vi "test Convert String To 9403 Module.vi"(8 "error in (no error)":errorcluster, 11 "TestCase in":refnum<class "RSI Module Unit Tests.lvclass">) -> (0 "error out":errorcluster, 3 "TestCase out":refnum<class "RSI Module Unit Tests.lvclass">)   [LabVIEW 2017, in "RSI Module Unit Tests.lvclass"]
uses:
  RSI Module Unit Tests.lvclass
  RSI Module/Module Models.ctl
  RSI Module/Slot Settings.ctl
  <vilib>/addons/_JKI Toolkits/VI Tester/TestCase.llb/TestCase.lvclass
  RSI Module/RSI Module.lvclass
  C:/Program Files (x86)/National Instruments/LabVIEW 2017/vi.lib/addons/_JKI Toolkits/VI Tester/TestCase.llb/TestCase.lvclass
panel:
  in  "xml string":string="<Object>\r\n<Name>RSI Module out</Name>\r\n<NumLevels>2</NumLevels>\r\n<Class>Modules.lvlib:9403.lvclass</Class>\r\n<Version>1.0.0.1</Version>\r\n<Version>1.0.0.21</Version>\r\n<Cluster>\r\n<Name>RSI Module.lvclass</Name>\r\n<NumElts>3</NumElts>\r\n<String>\r\n<Name>Module</Name>\r\n<Val>NI 9403</Val>\r\n</String>\r\n<Cluster>\r\n<Name>Slot Settings</Name>\r\n<NumElts>2</NumElts>\r\n<U32>\r\n<Name>Slot</Name>\r\n<Val>1</Val>\r\n</U32>\r\n<Boolean>\r\n<Name>EtherCAT?</Name>\r\n<Val>1</Val>\r\n</Boolean>\r\n</Cluster>\r\n<Cluster>\r\n<Name>Channels</Name>\r\n<NumElts>4</NumElts>\r\n<I32>\r\n<Name># Input Channels</Name>\r\n<Val>32</Val>\r\n</I32>\r\n<I32>\r\n<Name># Output Channels</Name>\r\n<Val>0</Val>\r\n</I32>\r\n<EW>\r\n<Name>Channel Type</Name>\r\n<Choice>Analog</Choice>\r\n<Choice>Digital</Choice>\r\n<Val>1</Val>\r\n</EW>\r\n<String>\r\n<Name>Units</Name>\r\n<Val></Val>\r\n</String>\r\n</Cluster>\r\n</Cluster>\r\n<Cluster>\r\n</Cluster>\r\n</Object>\r\n"
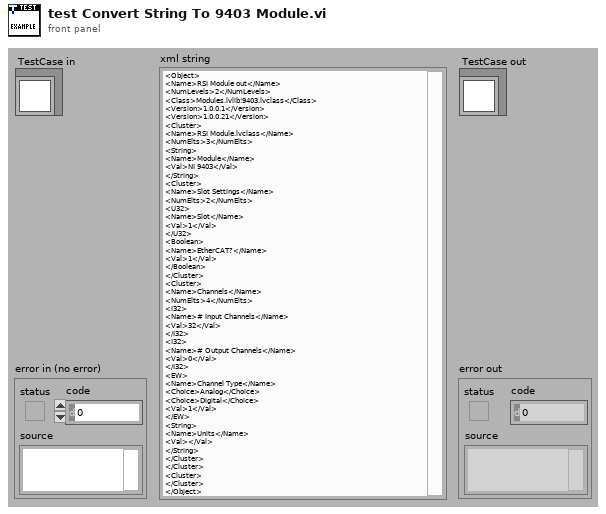
[diagram p1: front panel]
types:
  T1 = typedef "Modules.lvlib/RSI Module.lvclass/Slot Settings.ctl" = cluster{"Slot":u32, "EtherCAT?":bool}
  T2 = typedef "Modules.lvlib/RSI Module.lvclass/Module Models.ctl" = enum16{"Empty", "NI 9201", "NI 9203", "NI 9205", "NI 9206", "NI 9207", "NI 9208", "NI 9211", "NI 9212", "NI 9213", "NI 9214", "NI 9215", "NI 9217", "NI 9219", "NI 9220", "NI 9221", "NI 9222", "NI 9223", "NI 9225", "NI 9227", "NI 9229", "NI 9233", "NI 9234", "NI 9235", "NI 9236", "NI 9237", "NI 9239", "NI 9242", "NI 9244", "NI 9263", "NI 9264", "NI 9265", "NI 9266", "NI 9269", "NI 9375", "NI 9401", "NI 9402", "NI 9403", "NI 9411", "NI 9421", "NI 9422", "NI 9423", "NI 9425", "NI 9426", "NI 9435", "NI 9437", "NI 9472", "NI 9474", "NI 9475", "NI 9476", "NI 9477", "NI 9478", "NI 9481", "NI 9482", "NI 9485"}
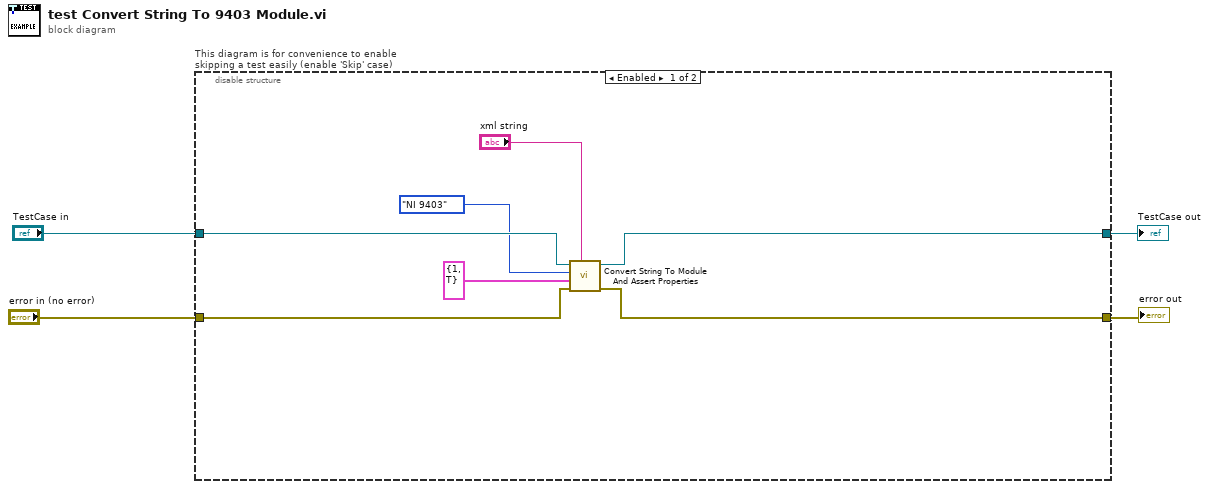
[diagram p0: block diagram]
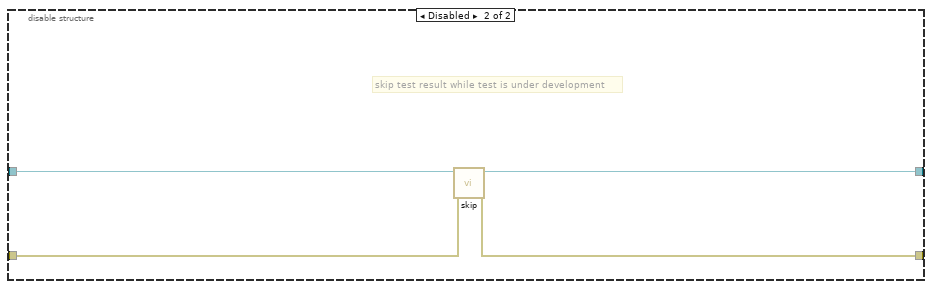
[diagram p2: hidden frame]
diagram:
  n1 = disable-structure "This diagram is for convenience to enable skipping a test easily (enable 'Skip' case)" shown="Enabled" {
    disable-tunnel: "TestCase in" -> [w11 w15]
    disable-tunnel: [w8 w13] -> w1
    disable-tunnel: [w9 w14] -> w3
    disable-tunnel: "error in (no error)" -> [w10 w12]
    frame Enabled {
      n2 = call "Convert String To Module And Assert Properties.vi"("String in"="xml string", "error in (no error)"=w10, "Slot Settings in"=T1 {"Slot"=1, "EtherCAT?"=TRUE}, "Module Model in"=Module_Models."NI 9403", "RSI Module Unit Tests in"=w11) -> ("error out"=w9:errorcluster, "RSI Module Unit Tests out"=w8:refnum<class "RSI Module Unit Tests.lvclass">)  [unwired: 4 in, 1 out]
    }
    frame Disabled {
      # "skip test result while test is under development"
      n3 = call <vilib>:"skip.vi"("error in (no error)"=w12, "TestCase in"=w15) -> ("error out"=w14:errorcluster, "TestCase out"=w13:refnum<class "RSI Module Unit Tests.lvclass">)  [unwired: 8 in]
    }
  }
  "error out" <- w3
  "TestCase out" <- w1
